vi "DAQLinescanVisualization.vi"(1 "Get/Set":bool, 2 "Visualization (input)":T1) -> (0 "Visualization (output)":T1)   [LabVIEW 2009]
uses:
  DAQLinescanVisualization.ctt
  <vilib>/vision/Image Controls.llb/IMAQ Image.ctl
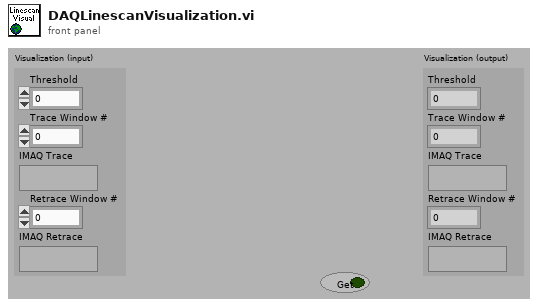
[diagram p1: front panel]
types:
  T1 = typedef "DAQLinescanVisualization.ctt" = cluster{"Threshold":u32, "Trace Window #":u32, "IMAQ Trace":T2, "Retrace Window #":u32, "IMAQ Retrace":T2}
  T2 = typedef "IMAQ Image.ctl" = refnum<image>
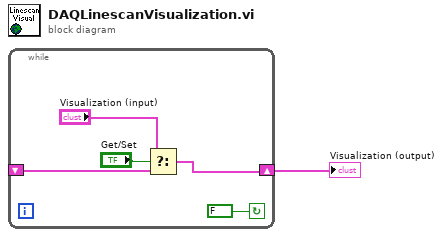
[diagram p0: block diagram]
diagram:
  n1 = while {
    shift-right: [w4] -> w1
    shift-left: _ -> [w5]
    stop <- FALSE continue-if-true
    n2 = Select(t="Visualization (input)", s="Get/Set", f=w5) -> (s? t:f=w4:T1)
  }
  "Visualization (output)" <- w1
